vi "Main.vi"(10 "VI":refnum<vi>, 11 "Module Admin":refnum<class "Delacor_lib_QMH_Module Admin.lvclass">) -> ()   [LabVIEW 2019, in "Full User Interface.lvlib"]
doc: "This template is based off of the Queued Message Handler design pattern and the Queued Message Handler project template that ships with LabVIEW.\n\nThe main difference is that the queue is private to this module and communication between modules is performed via Broadcast and Request events.\n\nRequest events are wrapped in public API methods and are handled in the Event Handling Loop (EHL) of this VI. Any module can register for Broadcast events sent by this module. The EHL generates messages based on user interface actions.\n\nThe Message Handling Loop (MHL) processes messages generated by the EHL, or by other messages. The messages are string values, so new messages can be added easily to the Message Cases case structure in the MHL. Each message cluster can also provide an optional value for Message Data, which is a variant that can be converted to whatever message-specific data is required.\n_____\nBased on DQMH Project Template 7.0.1.1316."
uses:
  Full User Interface.lvlib
  <vilib>/Delacor/Delacor QMH/Libraries/Module Admin_class/Delacor_lib_QMH_Module Admin.lvclass
  System.Windows.Forms
  Module Data--cluster.ctl
  Station Config.ctl
  Test Unit/UUT Result.ctl
  <vilib>/Test Bench Framework/Test Executive.lvlibp/TestEngine/TestEngine/TestEngine/Typedefs/Report General.ctl
  <vilib>/Test Bench Framework/Test Executive.lvlibp/TestEngine/TestEngine/TestEngine/Typedefs/TestEngine Cofiguration.ctl
  <vilib>/Test Bench Framework/Test Executive.lvlibp/TestEngine/TestEngine/TestEngine/Typedefs/Local Report Configuration.ctl
  <vilib>/Test Bench Framework/Test Executive.lvlibp/TestEngine/TestEngine/TestEngine/Report Format.ctl
  <vilib>/Test Bench Framework/Test Executive.lvlibp/TestEngine/TestEngine/TestEngine/Typedefs/Database Configuration.ctl
  <vilib>/Delacor/Delacor QMH/Libraries/Message Queue_class/Delacor_lib_QMH_Message Queue.lvclass/Delacor_lib_QMH_Message Queue.ctl
  Change Model Argument--cluster.ctl
  Stop Argument--cluster.ctl
  Launcher Test Unit Argument--cluster.ctl
  Exit Test Unit Argument--cluster.ctl
  Load Seq Argument--cluster.ctl
  Send UUT Result Argument--cluster.ctl
  Send User Message Argument--cluster.ctl
  <vilib>/Delacor/Delacor QMH/Libraries/Module Admin_class/Delacor_lib_QMH_Module Admin.lvclass/Delacor_lib_QMH_Module Admin.ctl
  <vilib>/Delacor/Delacor QMH/Libraries/Message Queue_class/Delacor_lib_QMH_Enqueue Message (Single).vi
  <vilib>/Delacor/Delacor QMH/Libraries/Module Admin_class/Delacor_lib_QMH_Get External Launch.vi
  d3b51c9b-000a-484a-be20-e9c62a2b2a8b.vi
  35dcfc0e-7b8d-49ca-9e41-10d6e4080697.vi
  e5b2156f-1627-4201-8ab9-82cd755b8a05.vi
  8e03fd14-8f50-4f43-832a-65f497bd3936.vi
  2ce45dc2-8b93-4d2c-831c-8eefbe131e90.vi
  7e8d7d5c-7c60-4828-99b6-0f7f76c7f789.vi
  <vilib>/Delacor/Delacor QMH/Libraries/Message Queue_class/Delacor_lib_QMH_Message Queue.lvclass
  Test Unit/Test Unit.lvlib
  <vilib>/Test Bench Framework/Test Executive.lvlibp/TestEngine/TestEngine/TestEngine/Test Engine.lvclass
  <vilib>/Test Bench Framework/Test Executive(API).lvlib
panel:
  in  "Panel":refnum<k24>(container)
  out "error out":errorcluster
  out "Status":string
  in  "Simulate MHL Error":bool
  in  "Simulate EHL Error":bool
types:
  T1 = typedef "Full User Interface.lvlib/Request Events--cluster.ctl" = cluster{"Stop Module":refnum<user-event>, "Show Panel":refnum<user-event>, "Hide Panel":refnum<user-event>, "Get Module Execution Status":refnum<user-event>, "Show Diagram":refnum<user-event>, "Launcher Test Unit":refnum<user-event>, "Exit Test Unit":refnum<user-event>, "Load Seq":refnum<user-event>, "Send UUT Result":refnum<user-event>, "Send User Message":refnum<user-event>, "Change Model":refnum<user-event>}
  T2 = typedef "Full User Interface.lvlib/Module Data--cluster.ctl" = cluster{"Status":string, "menu reference":refnum<k9>, "Key":string, "Config":T3, "UUT Result":refnum<user-event>, "Message":refnum<user-event>, "UserInfo":cluster{"Value":string, "Value":string}, "Configur":T4}
  T3 = typedef "Full User Interface.lvlib/Station Config.ctl" = map{string, map{i32, cluster{"SeqFilename":path, "NumberOfSocket":i32}}}
  T4 = typedef "Test Executive.lvlibp/Test Engine.lvlib/Test Engine.lvclass/TestEngine Cofiguration.ctl" = cluster{"Break on Failure":bool, "Automatically handle TestVI error":cluster{"Enable":bool, "Handle":enum16{"Termination test", "Ignore error"}}, "Local Report Configuration":T5, "Database Configuration":T7, "Ignore breakpoint":bool, "Filter Result":bool}
  T5 = typedef "Test Executive.lvlibp/Test Engine.lvlib/Test Engine.lvclass/Local Report Configuration.ctl" = cluster{"Report Folder Path":path, "Format":T6, "Disable":bool, "Build Date Folder?":bool}
  T6 = typedef "Test Executive.lvlibp/Test Engine.lvlib/Test Engine.lvclass/Report Format.ctl" = enum16{"Excel", "CSV(Tab)", "CSV(,)", "CSV(;)", "TEXT", "HTML"}
  T7 = typedef "Test Executive.lvlibp/Test Engine.lvlib/Test Engine.lvclass/Database Configuration.ctl" = cluster{"Connection String Expression":string, "Microsoft Data Link File":path, "Connection Type":enum16{"Use Connection String Expression", "Use Microsoft Data Link File"}, "Enable":bool}
  T8 = typedef "Full User Interface.lvlib/Change Model Argument--cluster.ctl" = cluster{"Model":string}
  T9 = enum32{"invalid lock state", "Not Locked", "Locked (No Password)", "Password-protected"}
  T10 = typedef "Full User Interface.lvlib/Stop Argument--cluster.ctl" = cluster{"Origin":string, "Exit via Stop Module Req?":bool, "Wait for Module to stop?":bool}
  T11 = typedef "Full User Interface.lvlib/Launcher Test Unit Argument--cluster.ctl" = cluster{"Checkbox":bool}
  T12 = typedef "Full User Interface.lvlib/Exit Test Unit Argument--cluster.ctl" = cluster{"Checkbox":bool}
  T13 = typedef "Full User Interface.lvlib/Load Seq Argument--cluster.ctl" = cluster{"Key":string}
  T14 = typedef "Full User Interface.lvlib/Send UUT Result Argument--cluster.ctl" = cluster{"UUT Result":T15, "Station":i32}
  T15 = typedef "Test Unit.lvlib/UUT Result.ctl" = cluster{"Station":i32, "Socket":i32, "DetailTestResult":string[][], "Report Path":path, "General":T16}
  T16 = typedef "Test Executive.lvlibp/Test Engine.lvlib/Test Engine.lvclass/Report General.ctl" = cluster{"Sequence Path":path, "Serial Number":string, "Test Date Time":timestamp, "UUT Status":string, "Faulty Item":string, "Seconds Executing":dbl}
  T17 = typedef "Full User Interface.lvlib/Send User Message Argument--cluster.ctl" = cluster{"Station ID":i32, "Socket":i32, "UserMessage":string, "MessageData":variant}
  T18 = enum32{"Invalid", "Standard", "Closed", "Hidden", "Minimized", "Maximized"}
  T19 = cluster{"Error":errorcluster, "Additional Information":string, "Module ID":i32, "Module Name":string}
  T20 = cluster{"Module ID":i32, "Origin":string, "Exit via Stop Module Req?":bool, "Wait for Module to stop?":bool}
  T21 = map{i32, cluster{"SeqFilename":path, "NumberOfSocket":i32}}
  T22 = cluster{"SeqFilename":path, "NumberOfSocket":i32}
  T23 = cluster{"Left":i32, "Top":i32, "Right":i32, "Bottom":i32}
  T24 = typedef "LVRectTypeDef.ctl" = cluster{"Left":i16, "Top":i16, "Right":i16, "Bottom":i16}
  T25 = cluster{"Error":errorcluster, "Additional Information":string, "Module Name":string}
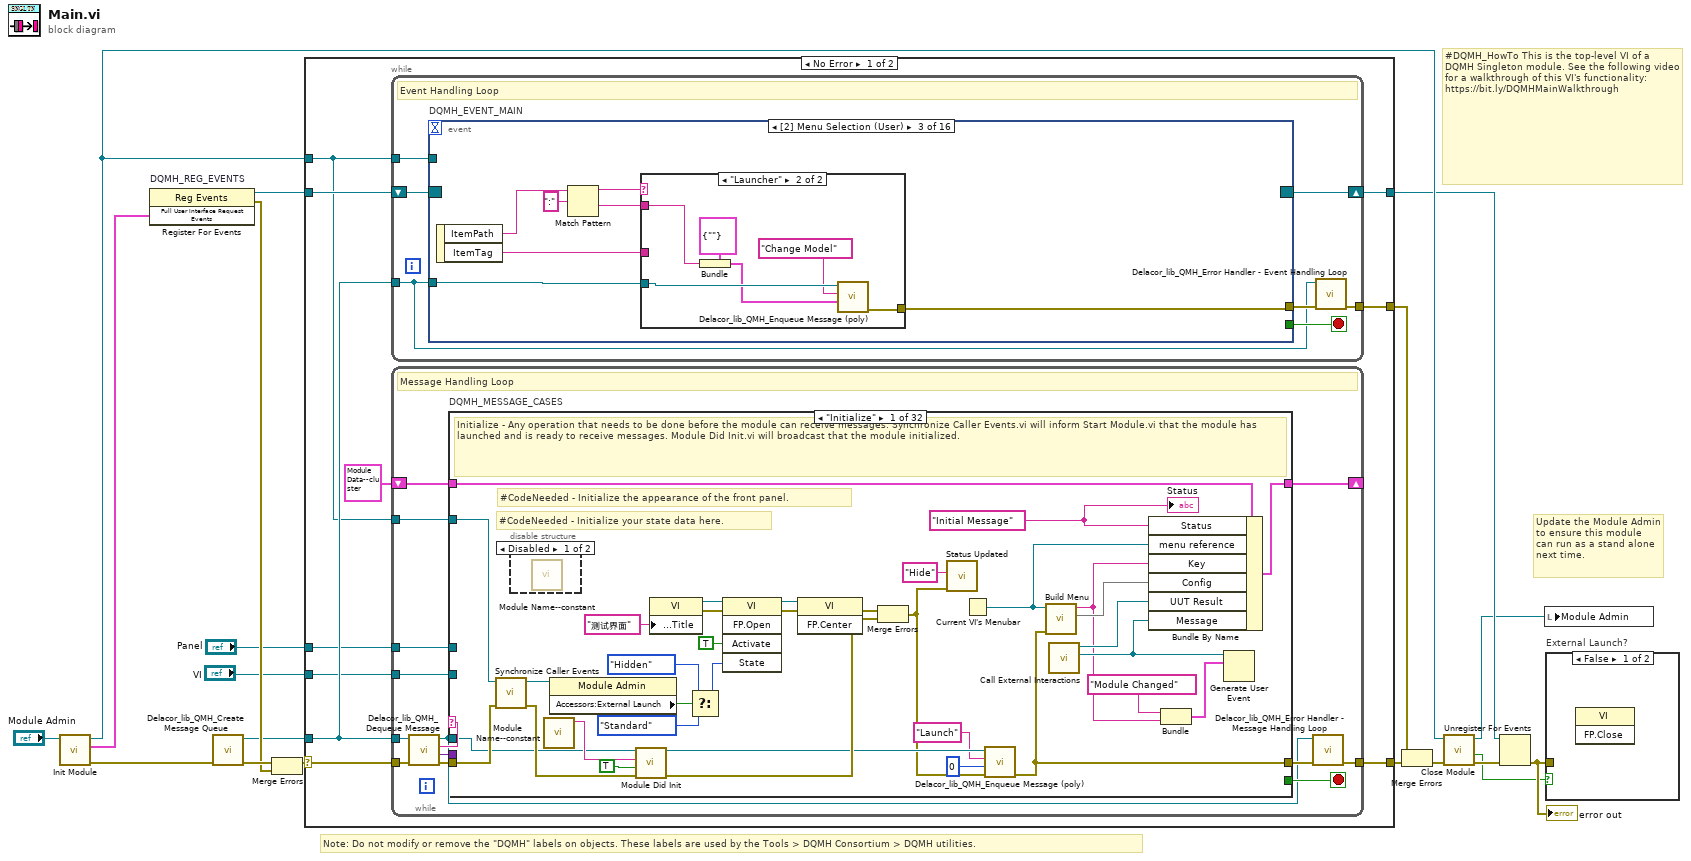
[diagram p0: block diagram]
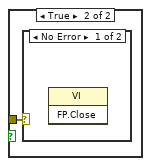
[diagram p2: hidden frame]
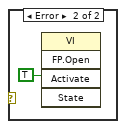
[diagram p3: hidden frame]
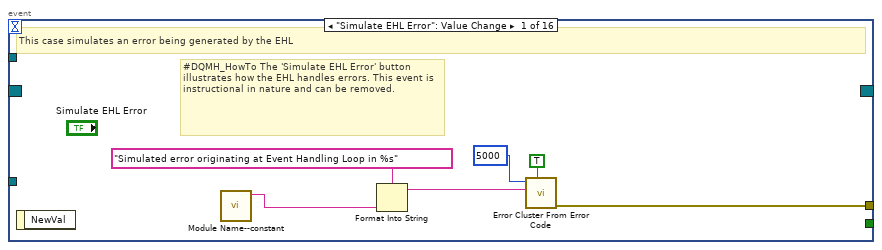
[diagram p4: hidden frame]
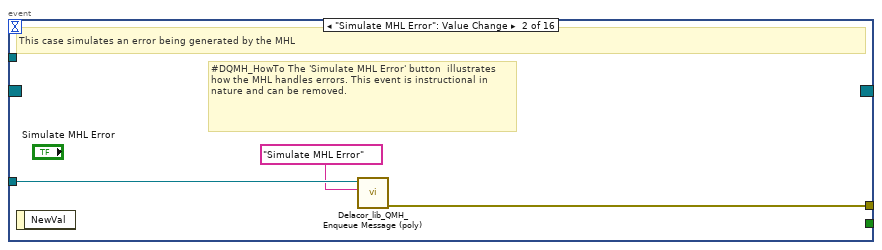
[diagram p5: hidden frame]
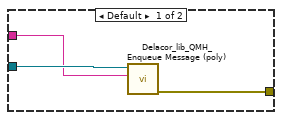
[diagram p6: hidden frame]
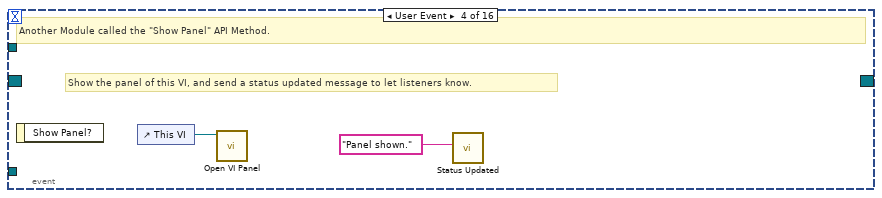
[diagram p7: hidden frame]
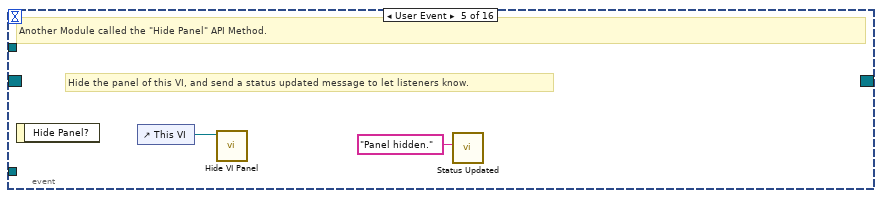
[diagram p8: hidden frame]
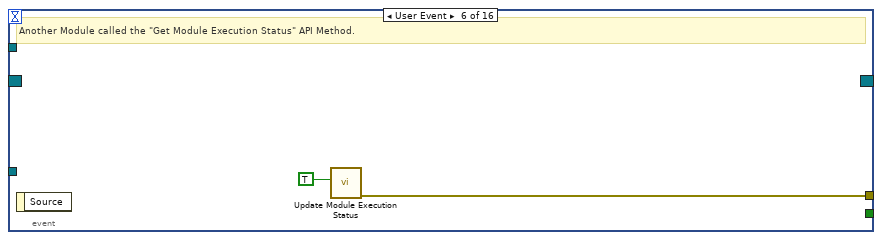
[diagram p9: hidden frame]
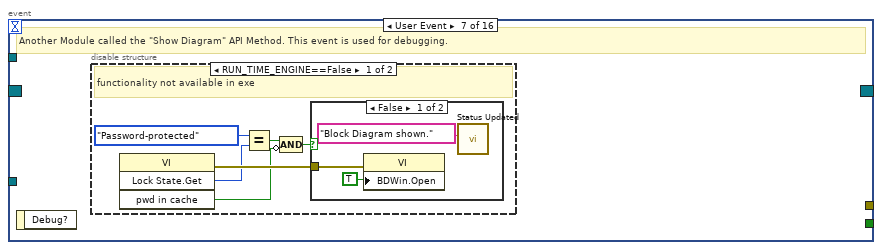
[diagram p10: hidden frame]
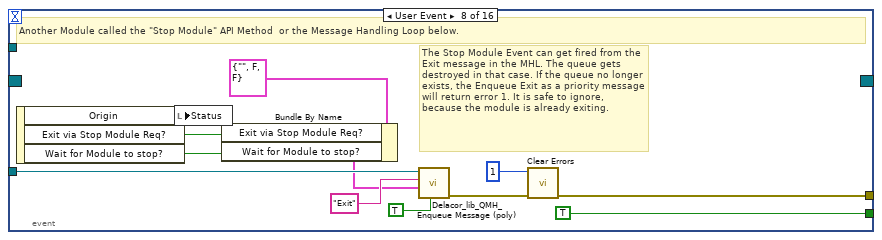
[diagram p13: hidden frame]
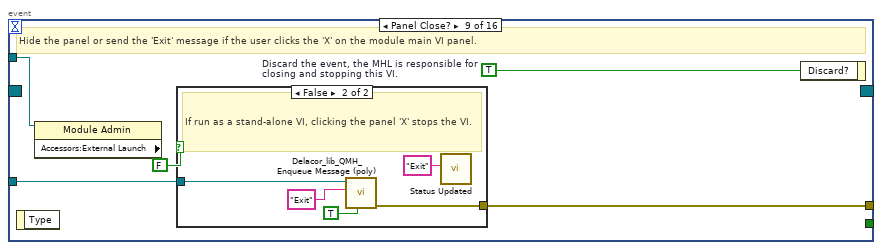
[diagram p14: hidden frame]
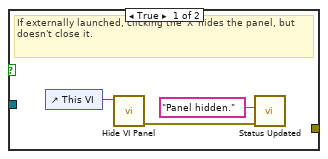
[diagram p15: hidden frame]
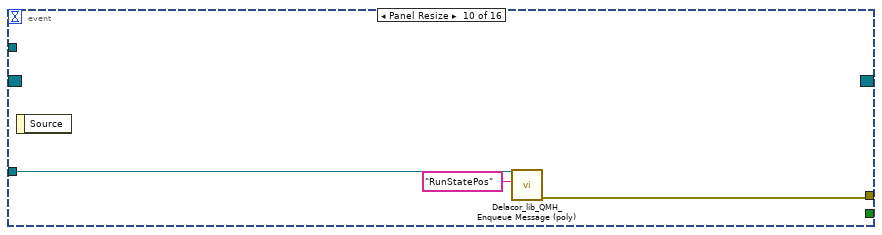
[diagram p16: hidden frame]
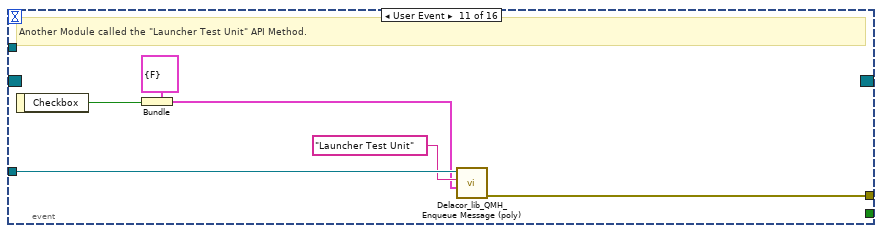
[diagram p17: hidden frame]
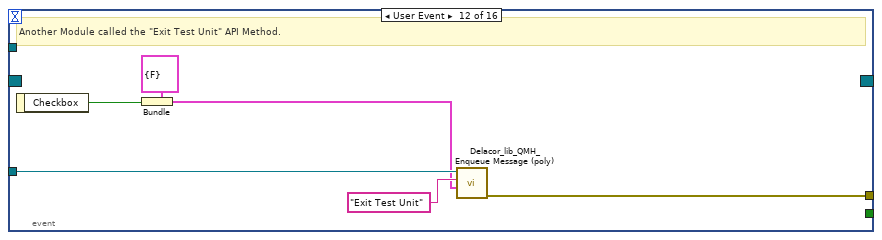
[diagram p18: hidden frame]
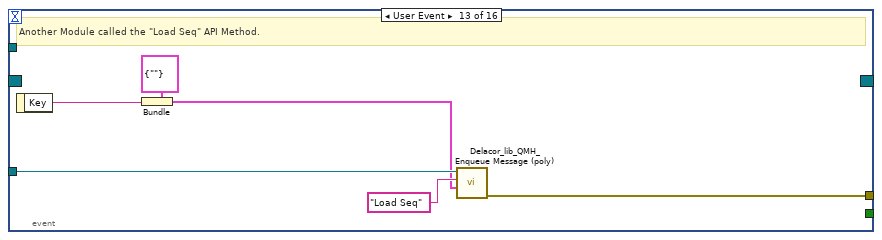
[diagram p19: hidden frame]
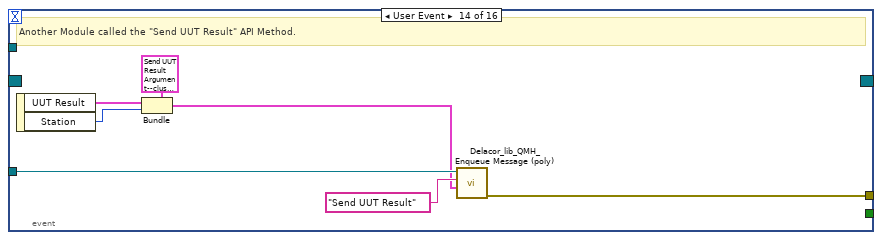
[diagram p20: hidden frame]
diagram:
  # "#DQMH_HowTo This is the top-level VI of a DQMH Singleton module. See the following video for a walkthrough of this VI's functionality: https://bit.ly/DQMHMainWalkthrough"
  # "Note: Do not modify or remove the \"DQMH\" labels on objects. These labels are used by the Tools > DQMH Consortium > DQMH utilities."
  # "Update the Module Admin to ensure this module can run as a stand alone next time."
  n1 = call "Init Module.vi"("Singleton Module Admin in"="Module Admin") -> ("error out"=w18:errorcluster, "Full User Interface Request Events"=w7:T1, "Singleton Module Admin out"=w10:refnum<class "Delacor_lib_QMH_Module Admin.lvclass">)  [unwired: 8 in]
  n2 = register-events "DQMH_REG_EVENTS"(w7) -> (reference out=w8:refnum<event-registration>, error out=w11:errorcluster)  [unwired: 2 in]
  n3 = call <vilib>:"Delacor_lib_QMH_Create Message Queue.vi"("error in"=w18) -> ("error out"=w13:errorcluster, "Message Queue"=w6:refnum<class "Delacor_lib_QMH_Message Queue.lvclass">)  [unwired: 9 in]
  n4 = Merge Errors(w13, w11) -> (w12:errorcluster)
  n5 = case shown="No Error" w12 {
    selector: w12 -> [w27 w536]
    tunnel: [w29 w535] -> w19
    tunnel: [w26 w534] -> w9
    tunnel: w8 -> [w24 w534]
    tunnel: w6 -> [w23 w529]
    tunnel: [w28 _] -> w16
    tunnel: w10 -> [w22 w530]
    tunnel: "Panel" -> [w21 _]
    tunnel: "VI" -> [w20 _]
    frame No Error {
      n6 = while {
        tunnel: w23 -> [w30]
        shift-right: [w33] -> w26
        shift-left: w24 -> [w34]
        tunnel: [w35] -> w28
        tunnel: w22 -> [w31]
        stop <- w32 stop-if-true
        # "Event Handling Loop"
        n7 = event "DQMH_EVENT_MAIN" shown="[2] Menu Selection (User)" {
          selector: w34 -> [_ _ _ _ _ _ _ _ _ _ _ _ _ _ _ _]
          dyn-events: [_ _ _ _ _ _ _ _ _ _ _ _ _ _ _ _] -> w33
          timeout: _ -> [_ _ _ _ _ _ _ _ _ _ _ _ _ _ _ _]
          tunnel: [_ _ _ _ _ _ _ TRUE ("Discard?") _ _ _ _ _ _ _ _] -> w32
          tunnel: w30 -> [_ w44 w52 _ _ _ _ w84 w91 w104 w110 w116 w122 w129 w138 w144]
          tunnel: [w42 w45 w50 _ _ w67 _ w87 w93 w103 w105 w111 w117 w123 w134 w139] -> w36
          tunnel: w31 -> [_ _ _ _ _ _ _ _ w90 _ _ _ _ _ _ _]
          event "Simulate EHL Error": Value Change {
            # "#DQMH_HowTo The 'Simulate EHL Error' button  illustrates how the EHL handles errors. This event is instructional in nature and can be removed."
            # "This case simulates an error being generated by the EHL"
            n8 = event-data() -> ()  [unwired: 1 in, 1 out]
            n9 = call "Module Name--constant.vi"() -> ("Module Name"=w39:string)  [unwired: 11 in]
            n10 = Format Into String(format string="Simulated error originating at Event Handling Loop in %s", w39) -> (resulting string=w40:string)  [unwired: 2 in, 1 out]
            n11 = call <vilib>:"Error Cluster From Error Code.vi"("show call chain? (False)"=TRUE, "error message (\"\")"=w40, "error code (0)"=5000) -> ("error out"=w42:errorcluster)  [unwired: 6 in]
          }
          event "Simulate MHL Error": Value Change {
            # "#DQMH_HowTo The 'Simulate MHL Error' button  illustrates how the MHL handles errors. This event is instructional in nature and can be removed."
            # "This case simulates an error being generated by the MHL"
            n12 = event-data() -> ()  [unwired: 1 in, 1 out]
            n13 = call-poly <vilib>:"Delacor_lib_QMH_Enqueue Message (poly).vi"("Message"="Simulate MHL Error", "Message Queue in"=w44) -> ("error out"=w45:errorcluster)  [unwired: 8 in, 1 out]
          }
          event Menu Selection (User) {
            n14 = event-data() -> ("ItemPath"=w49:string, "ItemTag"=w51:string)  [unwired: 1 in]
            n15 = Match Pattern(string=w49, regular expression=":") -> (before substring=w47:string, after substring=w46:string)  [unwired: 1 in, 2 out]
            n16 = case shown="\"Launcher\"" w47 {
              tunnel: w52 -> [w55 w60]
              tunnel: w51 -> [w54 _]
              tunnel: [w53 w61] -> w50
              tunnel: w46 -> [_ w57]
              frame Default {
                n17 = call-poly <vilib>:"Delacor_lib_QMH_Enqueue Message (poly).vi"("Message"=w54, "Message Queue in"=w55) -> ("error out"=w53:errorcluster)  [unwired: 8 in, 1 out]
              }
              frame "Launcher" {
                n18 = Bundle(cluster=T8 {"Model"=""} ("Change Model Argument"), "Model"=w57) -> (w56:T8)
                n19 = call-poly <vilib>:"Delacor_lib_QMH_Enqueue Message (poly).vi"("Message Data"=w56, "Message"="Change Model", "Message Queue in"=w60) -> ("error out"=w61:errorcluster)  [unwired: 7 in, 1 out]
              }
            }
          }
          event User Event {
            # "Show the panel of this VI, and send a status updated message to let listeners know."
            # "Another Module called the \"Show Panel\" API Method."
            n20 = event-data() -> ()  [unwired: 1 in, 1 out]
            n21 = control-ref of="This VI"() -> (w63:refnum<vi>)
            n22 = call "Open VI Panel.vi"("VI"=w63) -> ()  [unwired: 10 in, 1 out]
            n23 = call "Status Updated.vi"("Status"="Panel shown." ("format string")) -> ()  [unwired: 10 in, 1 out]
          }
          event User Event {
            # "Hide the panel of this VI, and send a status updated message to let listeners know."
            # "Another Module called the \"Hide Panel\" API Method."
            n24 = event-data() -> ()  [unwired: 1 in, 1 out]
            n25 = control-ref of="This VI"() -> (w65:refnum<vi>)
            n26 = call "Hide VI Panel.vi"("VI"=w65) -> ()  [unwired: 10 in, 1 out]
            n27 = call "Status Updated.vi"("Status"="Panel hidden." ("format string")) -> ()  [unwired: 10 in, 1 out]
          }
          event User Event {
            # "Another Module called the \"Get Module Execution Status\" API Method."
            n28 = event-data() -> ()  [unwired: 1 in, 1 out]
            n29 = call "Update Module Execution Status.vi"("Running?"=TRUE) -> ("error out"=w67:errorcluster)  [unwired: 10 in]
          }
          event User Event {
            # "Another Module called the \"Show Diagram\" API Method. This event is used for debugging."
            n30 = event-data() -> ()  [unwired: 1 in, 1 out]
            n31 = disable-structure shown="RUN_TIME_ENGINE==False" {
              frame condition #0 (active) {
                # "functionality not available in exe"
                n32 = invoke on="Invoke Node" class="VI" method="Lock State.Get"() -> (error out=w73:errorcluster, "Get Lock State"=w72:T9, "pwd in cache"=w69:bool)  [unwired: 4 in, 1 out]
                n33 = Equal?(x=T9."Password-protected", y=w72) -> (x = y?=w70:bool)
                n34 = Compound Arithmetic op=AND(w70, invert w69) -> (w68:bool)
                n35 = case shown="False" w68 {
                  tunnel: w73 -> [w76 _]
                  frame False {
                    n36 = property on="Property Node" class="VI"(error in=w76, "BDWin.Open"=TRUE ("Block Diagram Window:Open")) -> ()  [unwired: 1 in, 2 out]
                    n37 = call "Status Updated.vi"("Status"="Block Diagram shown." ("format string")) -> ()  [unwired: 10 in, 1 out]
                  }
                  frame True {
                    # "Password-protected VI, and the password is not in the cache. Do not show the diagram."
                  }
                }
              }
              frame condition #1 {
              }
            }
          }
          event User Event {
            # "The Stop Module Event can get fired from the Exit message in the MHL. The queue gets destroyed in that case. If the queue no longer exists, the Enqueue Exit as a priority message will return error 1. It is safe to ignore, because the module is already exiting."
            # "Another Module called the \"Stop Module\" API Method  or the Message Handling Loop below."
            n38 = event-data() -> ("Origin"=w83:string, "Exit via Stop Module Req?"=w79:bool, "Wait for Module to stop?"=w78:bool)  [unwired: 1 in]
            n39 = local write "Status"(w83) -> ()
            n40 = Bundle By Name(cluster=T10 {"Origin"="", "Exit via Stop Module Req?"=FALSE, "Wait for Module to stop?"=FALSE} ("Stop Argument"), "Exit via Stop Module Req?"=w79, "Wait for Module to stop?"=w78) -> (w77:T10)
            n41 = call-poly <vilib>:"Delacor_lib_QMH_Enqueue Message (poly).vi"("Priority Message? (F)"=TRUE, "Message Data"=w77, "Message"="Exit", "Message Queue in"=w84) -> ("error out"=w88:errorcluster)  [unwired: 6 in, 1 out]
            n42 = call <vilib>:"Clear Errors.vi"("error in (no error)"=w88, "specific error code to clear (0: all)"=1) -> ("error out"=w87:errorcluster)  [unwired: 4 in, 1 out]
          }
          event Panel Close? {
            w92 = TRUE  # Discard the event, the MHL is responsible for closing and stopping this VI.
            # "Hide the panel or send the 'Exit' message if the user clicks the 'X' on the module main VI panel."
            n43 = event-data() -> ()  [unwired: 1 in, 1 out]
            n44 = property on="Property Node" class="Module Admin" props=["Accessors:External Launch"](reference=w90) -> ()  [unwired: 1 in, 3 out]
            n45 = case shown="False" FALSE {
              tunnel: w91 -> [_ w100]
              tunnel: [_ w101] -> w93
              frame True {
                # "If externally launched, clicking the 'X' hides the panel, but doesn't close it."
                n46 = control-ref of="This VI"() -> (w96:refnum<vi>)
                n47 = call "Hide VI Panel.vi"("VI"=w96) -> ("error out"=w94:errorcluster)  [unwired: 10 in]
                n48 = call "Status Updated.vi"("error in"=w94, "Status"="Panel hidden." ("format string")) -> ()  [unwired: 9 in, 1 out]
              }
              frame False {
                # "If run as a stand-alone VI, clicking the panel 'X' stops the VI."
                n49 = call-poly <vilib>:"Delacor_lib_QMH_Enqueue Message (poly).vi"("Priority Message? (F)"=TRUE, "Message"="Exit", "Message Queue in"=w100) -> ("error out"=w101:errorcluster)  [unwired: 7 in, 1 out]
                n50 = call "Status Updated.vi"("Status"="Exit") -> ()  [unwired: 10 in, 1 out]
              }
            }
            n51 = event-data ("Event Filter Node")("Discard?"=w92) -> ()  [unwired: 1 in, 1 out]
          }
          event Panel Resize {
            n52 = event-data() -> ()  [unwired: 1 in, 1 out]
            n53 = call-poly <vilib>:"Delacor_lib_QMH_Enqueue Message (poly).vi"("Message"="RunStatePos", "Message Queue in"=w104) -> ("error out"=w103:errorcluster)  [unwired: 8 in, 1 out]
          }
          event User Event {
            # "Another Module called the \"Launcher Test Unit\" API Method."
            n54 = event-data() -> ("Checkbox"=w106:bool)  [unwired: 1 in]
            n55 = Bundle(cluster=T11 {"Checkbox"=FALSE} ("Launcher Test Unit Argument"), "Checkbox"=w106) -> (w107:T11)
            n56 = call-poly <vilib>:"Delacor_lib_QMH_Enqueue Message (poly).vi"("Message Data"=w107, "Message"="Launcher Test Unit", "Message Queue in"=w110) -> ("error out"=w105:errorcluster)  [unwired: 7 in, 1 out]
          }
          event User Event {
            # "Another Module called the \"Exit Test Unit\" API Method."
            n57 = event-data() -> ("Checkbox"=w112:bool)  [unwired: 1 in]
            n58 = Bundle(cluster=T12 {"Checkbox"=FALSE} ("Exit Test Unit Argument"), "Checkbox"=w112) -> (w113:T12)
            n59 = call-poly <vilib>:"Delacor_lib_QMH_Enqueue Message (poly).vi"("Message Data"=w113, "Message"="Exit Test Unit", "Message Queue in"=w116) -> ("error out"=w111:errorcluster)  [unwired: 7 in, 1 out]
          }
          event User Event {
            # "Another Module called the \"Load Seq\" API Method."
            n60 = event-data() -> ("Key"=w118:string)  [unwired: 1 in]
            n61 = Bundle(cluster=T13 {"Key"=""} ("Load Seq Argument"), "Key"=w118) -> (w119:T13)
            n62 = call-poly <vilib>:"Delacor_lib_QMH_Enqueue Message (poly).vi"("Message Data"=w119, "Message"="Load Seq", "Message Queue in"=w122) -> ("error out"=w117:errorcluster)  [unwired: 7 in, 1 out]
          }
          event User Event {
            # "Another Module called the \"Send UUT Result\" API Method."
            n63 = event-data() -> ("UUT Result"=w125:T15, "Station"=w124:i32)  [unwired: 1 in]
            n64 = Bundle(cluster=T14 {"UUT Result"={"Station"=0, "Socket"=0, "DetailTestResult"=[], "Report Path"=path "", "General"={"Sequence Path"=path "", "Serial Number"="", "Test Date Time"=timestamp(0 s since 1904-01-01), "UUT Status"="", "Faulty Item"="", "Seconds Executing"=0.0}}, "Station"=0} ("Send UUT Result Argument"), "UUT Result"=w125, "Station"=w124) -> (w126:T14)
            n65 = call-poly <vilib>:"Delacor_lib_QMH_Enqueue Message (poly).vi"("Message Data"=w126, "Message"="Send UUT Result", "Message Queue in"=w129) -> ("error out"=w123:errorcluster)  [unwired: 7 in, 1 out]
          }
          event User Event {
            # "Another Module called the \"Send User Message\" API Method."
            n66 = event-data() -> ("Station ID"=w133:i32, "Socket"=w132:i32, "UserMessage"=w131:string, "MessageData"=w130:variant)  [unwired: 1 in]
            n67 = Bundle(cluster=T17 {"Station ID"=0, "Socket"=0, "UserMessage"="", "MessageData"=variant(cluster{"Socket":i32, "UserMessage":string, "MessageData":variant} {"Socket"=0, "UserMessage"="", "MessageData"=variant})} ("Send User Message Argument"), "Station ID"=w133, "Socket"=w132, "UserMessage"=w131, "MessageData"=w130) -> (w135:T17)
            n68 = call-poly <vilib>:"Delacor_lib_QMH_Enqueue Message (poly).vi"("Message Data"=w135, "Message"="Send User Message", "Message Queue in"=w138) -> ("error out"=w134:errorcluster)  [unwired: 7 in, 1 out]
          }
          event User Event {
            # "Another Module called the \"Change Model\" API Method."
            n69 = event-data() -> ("Model"=w140:string)  [unwired: 1 in]
            n70 = Bundle(cluster=T8 {"Model"=""} ("Change Model Argument"), "Model"=w140) -> (w141:T8)
            n71 = call-poly <vilib>:"Delacor_lib_QMH_Enqueue Message (poly).vi"("Message Data"=w141, "Message"="Change Model", "Message Queue in"=w144) -> ("error out"=w139:errorcluster)  [unwired: 7 in, 1 out]
          }
        }
        n72 = call-dynamic "Delacor_lib_QMH_Error Handler - Event Handling Loop.vi"("error in"=w36, "Message Queue in"=w30) -> ("dup error in"=w35:errorcluster)  [unwired: 8 in, 1 out]
      }
      n73 = while {
        tunnel: w23 -> [w147]
        shift-right: [w155] -> _
        shift-left: T2 {"Status"="", "menu reference"=refnum, "Key"="", "Config"={}, "UUT Result"=refnum, "Message"=refnum, "UserInfo"={"Value"="", "Value"=""}, "Configur"={"Break on Failure"=FALSE, "Automatically handle TestVI error"={"Enable"=FALSE, "Handle"=enum."Termination test"}, "Local Report Configuration"={"Report Folder Path"=path "", "Format"=enum."Excel", "Disable"=FALSE, "Build Date Folder?"=FALSE}, "Database Configuration"={"Connection String Expression"="", "Microsoft Data Link File"=path "", "Connection Type"=enum."Use Connection String Expression", "Enable"=FALSE}, "Ignore breakpoint"=FALSE, "Filter Result"=FALSE}} ("Data Cluster") -> [w156]
        tunnel: w27 -> [w158]
        tunnel: [w150] -> w29
        tunnel: w22 -> [w151]
        tunnel: w21 -> [w146]
        tunnel: w20 -> [w145]
        stop <- w154 stop-if-true
        # "Message Handling Loop"
        n74 = call-dynamic "Delacor_lib_QMH_Dequeue Message.vi"("error in"=w158, "Message Queue in"=w147) -> ("error out"=w157:errorcluster, "Message Data"=w152:variant, "Message"=w153:string, "Message Queue out"=w148:refnum<class "Delacor_lib_QMH_Message Queue.lvclass">)  [unwired: 6 in]
        n75 = case "DQMH_MESSAGE_CASES" shown="\"Initialize\"" w153 {
          selector: w153 -> [_ _ _ _ _ _ _ _ _ _ _ _ _ _ _ _ _ _ _ _ _ _ _ _ _ _ _ _ _ _ _ w524]
          tunnel: w148 -> [w173 _ w208 w228 w262 _ _ w289 w304 _ _ _ _ _ _ _ _ _ _ w409 _ _ _ _ _ _ _ _ _ w486 w512 _]
          tunnel: w157 -> [w190 w194 w207 w229 w264 w272 w279 w296 w308 w310 w326 w344 w354 w357 w362 w377 w392 w398 w404 w408 w424 w434 w448 w457 w460 w468 w471 w473 w482 w493 w518 w527]
          tunnel: [w170 w194 w206 w226 w260 w269 w276 w288 w305 w309 w318 w343 w353 w356 w361 w376 w391 w399 w403 w419 w423 w433 w447 w456 w459 w468 w471 w473 w481 w489 w513 w528] -> w149
          tunnel: w156 -> [w181 w193 w202 w222 w265 w268 w275 w292 w307 w313 w325 w339 w350 w355 w360 w375 w390 w396 w402 w418 w422 w432 w446 w455 w458 w467 w470 w472 w479 w488 w500 w525]
          tunnel: [w180 w193 w202 w222 w265 w266 w273 w291 w307 w313 w325 w339 w350 w355 w360 w375 w390 w395 w402 w418 w422 w432 w446 w455 w458 w467 w470 w472 w479 w488 w500 w525] -> w155
          tunnel: [_ _ _ _ _ _ _ _ _ _ _ _ _ _ _ _ _ _ _ _ _ _ _ _ _ _ _ _ _ _ w511 _] -> w154
          tunnel: w152 -> [_ _ w205 w236 _ _ _ w295 _ _ w323 w342 w352 _ _ _ _ _ _ _ _ w431 w445 w454 _ _ _ _ _ w487 w510 _]
          tunnel: w151 -> [w182 _ _ _ _ _ _ _ _ _ _ _ _ _ _ _ _ _ _ _ _ _ _ _ _ _ _ _ _ w485 w505 _]
          tunnel: w146 -> [_ _ _ w232 _ _ _ _ _ _ _ _ _ _ _ w373 w386 _ _ _ _ _ _ _ _ _ _ _ _ _ _ _]
          tunnel: w145 -> [_ _ _ _ _ _ _ _ _ _ _ _ _ _ _ _ _ _ _ _ w421 _ _ _ _ _ _ _ _ _ _ _]
          frame "Initialize" {
            w176 = "Initial Message" ("Initial Message")
            # "#CodeNeeded - Initialize the appearance of the front panel."
            # "#CodeNeeded - Initialize your state data here."
            # "Initialize - Any operation that needs to be done before the module can receive messages. Synchronize Caller Events.vi will inform Start Module.vi that the module has launched and is ready to receive messages. Module Did Init.vi will broadcast that the module initialized."
            n76 = call "Synchronize Caller Events.vi"("error in"=w190, "Singleton Module Admin in"=w182) -> ("error out"=w189:errorcluster, "Singleton Module Admin out"=w177:refnum<class "Delacor_lib_QMH_Module Admin.lvclass">)  [unwired: 8 in]
            n77 = disable-structure shown="Disabled" {
              frame Disabled {
                n78 = call "Module Name--constant.vi"() -> ()  [unwired: 11 in, 1 out]
              }
              frame Enabled {
              }
            }
            n79 = call "Module Name--constant.vi"() -> ("Module Name"=w178:string)  [unwired: 11 in]
            n80 = property on="Property Node" class="Module Admin"(reference=w177) -> ("Accessors:External Launch"=w186:bool)  [unwired: 1 in, 2 out]
            n81 = call "Module Did Init.vi"("error in"=w189, "Initialized?"=TRUE, "Origin"=w178) -> ("error out"=w174:errorcluster)  [unwired: 8 in]
            n82 = property on="Property Node" class="VI"("Front Panel.Title"="测试界面" ("Front Panel Window:Title")) -> (reference out=w188:refnum<vi>, error out=w192:errorcluster)  [unwired: 2 in]
            n83 = Select(t=T18."Hidden" ("State"), s=w186, f=T18."Standard" ("State")) -> (s? t:f=w183:T18)
            n84 = invoke on="Invoke Node" class="VI" method="FP.Open"(reference=w188, error in=w192, "Activate"=TRUE ("Activate?"), "State"=w183) -> (reference out=w187:refnum<vi>, error out=w191:errorcluster)  [unwired: 1 in, 3 out]
            n85 = invoke on="Invoke Node" class="VI" method="FP.Center"(reference=w187, error in=w191) -> (error out=w175:errorcluster)  [unwired: 1 in, 2 out]
            n86 = Merge Errors(w175, w174) -> (w164:errorcluster)
            n87 = call "Status Updated.vi"("error in"=w164, "Status"="Hide") -> ()  [unwired: 9 in, 1 out]
            n88 = Current VI's Menubar() -> (w169:refnum<k9>)
            n89 = call-poly <vilib>:"Delacor_lib_QMH_Enqueue Message (poly).vi"("error in"=w164, "Message Data"=0, "Message"="Launch", "Message Queue in"=w173) -> ("error out"=w170:errorcluster)  [unwired: 6 in, 1 out]
            n90 = call "Build Menu.vi"("error in (no error)"=w170, "menu reference"=w169) -> ("Station Config"=w166:T3, "element"=w160:string)  [unwired: 7 in, 1 out]
            n91 = call "Call External Interactions.vi"() -> ("Message"=w161:refnum<user-event>, "UUT Result"=w165:refnum<user-event>)  [unwired: 9 in, 1 out]
            n92 = Bundle By Name(cluster=w181, "Status"=w176, "menu reference"=w169, "Key"=w160, "Config"=w166, "UUT Result"=w165, "Message"=w161) -> (w180:T2)
            n93 = Bundle("Msg"="Module Changed", "element"=w160) -> (w162:cluster{"Msg":string, "element":string})  [unwired: 1 in]
            n94 = Generate User Event(user event=w161, event data cluster=w162) -> ()  [unwired: 2 in, 2 out]
            "Status" <- w176
          }
          frame "---Module Specific---" {
            # "Separator -- The following cases handle messages specific to this Module."
          }
          frame "Launch" {
            # "Separator -- The following cases handle messages specific to this Module."
            n95 = Variant To Data(type=0, Variant=w205) -> (data=w197:i32)  [unwired: 1 in, 1 out]
            n96 = Unbundle By Name(w202) -> ("Config"=w201:T3, "Key"=w200:string)
            n97 = Look In Map(map=w201, key=w200) -> (key not found?=w199:bool, value=w198:T21)  [unwired: 1 in]
            n98 = Equal To 0?(x=w197) -> (x = 0?=w203:bool)
            n99 = Look In Map(map=w198, key=w197) -> (value=w196:T22)  [unwired: 1 in, 1 out]
            n100 = Unbundle(w196) -> ("NumberOfSocket"=w195:i32)  [unwired: 1 out]
            n101 = case shown="False" w199 {
              tunnel: w208 -> [w213 _]
              tunnel: w207 -> [w212 w214]
              tunnel: [w211 w214] -> w206
              tunnel: w203 -> [w210 _]
              tunnel: w195 -> [w209 _]
              frame False {
                n102 = call "Launch Test Unit.vi"("error in"=w212, "Init Module ID"=w210, "Number of socket"=w209, "Message Queue"=w213) -> ("error out"=w211:errorcluster)  [unwired: 7 in]
              }
              frame True {
              }
            }
          }
          frame "Set Paraent" {
            # "Separator -- The following cases handle messages specific to this Module."
            n103 = Unbundle By Name(w222) -> ("Config"=w223:T3, "Key"=w219:string)
            n104 = Variant To Data(type=cluster{"Module ID":i32, "This VI":refnum<vi>} {"Module ID"=0, "This VI"=refnum} ("output cluster"), Variant=w236) -> (data=w234:cluster{"Module ID":i32, "This VI":refnum<vi>})  [unwired: 1 in, 1 out]
            n105 = Look In Map(map=w223, key=w219) -> (value=w221:T21)  [unwired: 1 in, 1 out]
            n106 = Unbundle(w234) -> ("Module ID"=w217:i32, "This VI"=w233:refnum<vi>)
            n107 = Collection Size(1:w221) -> (0:w220:i32)
            n108 = Equal?(x=w217, y=w220) -> (x = y?=w227:bool)
            n109 = call "Get Win Handle.vi"(".NET Refnum in"=w232) -> ("Bounds"=w224:T23, "ToInt32"=w225:i32)  [unwired: 7 in, 2 out]
            n110 = call "Find Windows.vi"("VI reference"=w233) -> ("hWnd"=w231:u32)  [unwired: 9 in, 1 out]
            n111 = Format Into String(format string="Test Unit %d", w217) -> (resulting string=w216:string)  [unwired: 2 in, 1 out]
            n112 = To Long Integer(number=w231) -> (32bit integer=w230:i32)
            n113 = call "Module Did Init.vi"("Initialized?"=TRUE, "Origin"=w216) -> ()  [unwired: 9 in, 1 out]
            n114 = call "SetParent.vi"("hWndNewParent"=w225, "hWndChild"=w230) -> ()  [unwired: 8 in, 2 out]
            n115 = case shown="True" w227 {
              tunnel: w229 -> [w241 w256]
              tunnel: w228 -> [w240 w245]
              tunnel: [w239 w243] -> w226
              tunnel: w225 -> [_ w259]
              tunnel: w224 -> [_ w258]
              tunnel: w217 -> [w237 _]
              tunnel: w219 -> [_ w250]
              frame False {
                n116 = call-poly <vilib>:"Delacor_lib_QMH_Enqueue Message (poly).vi"("error in"=w241, "Message Data"=w237, "Message"="Launch", "Message Queue in"=w240) -> ("error out"=w239:errorcluster)  [unwired: 6 in, 1 out]
              }
              frame True {
                n117 = call "Stall Data Flow.vim"("value in"=w256, "milliseconds to wait"=u32 100) -> ("value out"=w247:errorcluster)  [unwired: 1 out]
                n118 = call "TileWindows.vi"("Front Panel Window:Panel Bounds"=w258, "error in (no error)"=w247, "hWnd"=w259) -> ("error out"=w257:errorcluster)  [unwired: 8 in]
                n119 = call "Stall Data Flow.vim"("value in"=w257, "milliseconds to wait"=u32 100) -> ("value out"=w252:errorcluster)  [unwired: 1 out]
                n120 = call "TitleWindows.vi"("dont initi"=TRUE, "error in"=w252, "TitleWindows"=TRUE, "Module ID"=-1) -> ("error out"=w244:errorcluster)  [unwired: 7 in]
                n121 = call "Stall Data Flow.vim"("value in"=w244, "milliseconds to wait"=u32 100) -> ("value out"=w249:errorcluster)  [unwired: 1 out]
                n122 = call-poly <vilib>:"Delacor_lib_QMH_Enqueue Message (poly).vi"("error in"=w244, "Message"="SetTestUnitConfig", "Message Queue in"=w245) -> ("error out"=w243:errorcluster)  [unwired: 7 in, 1 out]
                n123 = call "Load Seq.vi"("error in"=w249, "Key"=w250) -> ()  [unwired: 9 in, 1 out]
              }
            }
          }
          frame "TestUnitConfig" {
            n124 = call "Config.vi"("Error In"=w264) -> ("Error Out"=w263:errorcluster)  [unwired: 10 in]
            n125 = call-poly <vilib>:"Delacor_lib_QMH_Enqueue Message (poly).vi"("error in"=w263, "Message"="SetTestUnitConfig", "Message Queue in"=w262) -> ("error out"=w260:errorcluster)  [unwired: 7 in, 1 out]
          }
          frame "SetTestUnitConfig" {
            n126 = call "Get Config.vi"("error in (no error)"=w272) -> ("error out"=w271:errorcluster, "Configur"=w267:T4)  [unwired: 9 in]
            n127 = Bundle By Name(cluster=w268, "Configur"=w267) -> (w266:T2)
            n128 = call "Cofiguration.vi"("error in"=w271, "TestEngine Cofiguration"=w267, "Module ID"=-1) -> ("error out"=w269:errorcluster)  [unwired: 8 in]
          }
          frame "StationConfig" {
            n129 = call "Station Config.vi"("error IO"=w279) -> ("error IO 2"=w277:errorcluster)  [unwired: 10 in]
            n130 = Unbundle By Name(w275) -> ("menu reference"=w278:refnum<k9>)
            n131 = call "ReBuild Menu.vi"("error in (no error)"=w277, "menu reference"=w278) -> ("error out"=w276:errorcluster, "Station Config"=w274:T3)  [unwired: 8 in]
            n132 = Bundle By Name(cluster=w275, "Config"=w274) -> (w273:T2)
          }
          frame "Change Model" {
            n133 = Variant To Data(type=T8 {"Model"=""} ("Change Model Argument"), Variant=w295) -> (data=w284:T8)  [unwired: 1 in, 1 out]
            n134 = Unbundle By Name(w292) -> ("menu reference"=w294:refnum<k9>, "Message"=w283:refnum<user-event>)
            n135 = Unbundle By Name(w284) -> ("Model"=w281:string)
            n136 = call "Select Config.vi"("item tag"=w281, "menu reference"=w294) -> ("error out"=w293:errorcluster)  [unwired: 9 in]
            n137 = Bundle("Msg"="Module Changed", "Model"=w281) -> (w280:cluster{"Msg":string, "Model":string})  [unwired: 1 in]
            n138 = Generate User Event(user event=w283, event data cluster=w280) -> ()  [unwired: 2 in, 2 out]
            n139 = call "Get Station Config.vi"() -> ("Station Config"=w286:T3)  [unwired: 10 in, 1 out]
            n140 = Bundle By Name(cluster=w292, "Key"=w281, "Config"=w286) -> (w291:T2)
            n141 = Merge Errors(w293, w296) -> (w290:errorcluster)
            n142 = for {
              tunnel: w289 -> [w301]
              shift-right: [w298] -> w288
              shift-left: w290 -> [w302]
              tunnel: string[] ["Exit Test Unit", "Launcher Test Unit"] -> [w299] mode=indexing
              n143 = call-poly <vilib>:"Delacor_lib_QMH_Enqueue Message (poly).vi"("error in"=w302, "Message"=w299, "Message Queue in"=w301) -> ("error out"=w300:errorcluster)  [unwired: 7 in, 1 out]
              n144 = call "Stall Data Flow.vim"("value in"=w300, "milliseconds to wait"=u32 100) -> ("value out"=w298:errorcluster)  [unwired: 1 out]
            }
          }
          frame "Launcher Test Unit" {
            n145 = call-poly <vilib>:"Delacor_lib_QMH_Enqueue Message (poly).vi"("error in"=w308, "Message Data"=0, "Message"="Launch", "Message Queue in"=w304) -> ("error out"=w305:errorcluster)  [unwired: 6 in, 1 out]
          }
          frame "Exit Test Unit" {
            # "#CodeNeeded\n1. Configure this Message Case for handling the \"Exit Test Unit\" message.\n2. Delete or edit this label when done."
            n146 = call "Stop Module.vi"("error in"=w310, "Wait for Module to stop? (F)"=TRUE, "Module ID"=-1) -> ("error out"=w309:errorcluster)  [unwired: 8 in]
          }
          frame "Load Seq" {
            n147 = Variant To Data(error in=w326, type=T13 {"Key"=""} ("Load Seq Argument"), Variant=w323) -> (data=w321:T13, error out=w324:errorcluster)
            n148 = Unbundle By Name(w321) -> ("Key"=w316:string)
            n149 = call "Get Station Config.vi"() -> ("Station Config"=w320:T3)  [unwired: 10 in, 1 out]
            n150 = Look In Map(map=w320, key=w316) -> (value=w319:T21)  [unwired: 1 in, 1 out]
            n151 = for {
              tunnel: w319 -> [w334] mode=indexing
              shift-right: [w328] -> w317
              shift-left: _ -> [w327]
              n152 = Unbundle(w334) -> ("Station"=w333:i32, "value"=w332:T22)
              n153 = Unbundle(w332) -> ("SeqFilename"=w330:path)  [unwired: 1 out]
              n154 = Increment(x=w333) -> (x+1=w331:i32)
              n155 = call "Load Sequence.vi"("error in"=w327, "Sequence"="Main_Sequence", "File Pathname"=w330, "Module ID"=w331) -> ("error out"=w328:errorcluster)  [unwired: 7 in]
            }
            n156 = Format Into String(format string="Switch Product %s", w316) -> (resulting string=w314:string)  [unwired: 2 in, 1 out]
            n157 = call "Status Updated.vi"("Status"=w314) -> ()  [unwired: 10 in, 1 out]
            n158 = Merge Errors(w317, w324) -> (w318:errorcluster)
          }
          frame "Send UUT Result" {
            n159 = Variant To Data(error in=w344, type=T14 {"UUT Result"={"Station"=0, "Socket"=0, "DetailTestResult"=[], "Report Path"=path "", "General"={"Sequence Path"=path "", "Serial Number"="", "Test Date Time"=timestamp(0 s since 1904-01-01), "UUT Status"="", "Faulty Item"="", "Seconds Executing"=0.0}}, "Station"=0} ("Send UUT Result Argument"), Variant=w342) -> (data=w340:T14, error out=w343:errorcluster)
            n160 = Unbundle By Name(w340) -> ("UUT Result"=w336:T15, "Station"=w337:i32)
            n161 = Unbundle By Name(w339) -> ("UUT Result"=w338:refnum<user-event>)
            n162 = Bundle("Station"=w337, "UUT Result"=w336) -> (w335:cluster{"Station":i32, "UUT Result":T15})  [unwired: 1 in]
            n163 = Generate User Event(user event=w338, event data cluster=w335) -> ()  [unwired: 2 in, 2 out]
          }
          frame "Send User Message" {
            n164 = Variant To Data(error in=w354, type=T17 {"Station ID"=0, "Socket"=0, "UserMessage"="", "MessageData"=variant(cluster{"Socket":i32, "UserMessage":string, "MessageData":variant} {"Socket"=0, "UserMessage"="", "MessageData"=variant})} ("Send User Message Argument"), Variant=w352) -> (data=w348:T17, error out=w353:errorcluster)
            n165 = Unbundle By Name(w350) -> ("Message"=w349:refnum<user-event>)
            n166 = To Variant(anything=w348) -> (Variant=w347:variant)
            n167 = Bundle("Msg"="Client Message", "Variant"=w347) -> (w345:cluster{"Msg":string, "Variant":variant})  [unwired: 1 in]
            n168 = Generate User Event(user event=w349, event data cluster=w345) -> ()  [unwired: 2 in, 2 out]
          }
          frame "---Copy This Frame---" {
            # "Duplicate this frame when creating new messages.  Change this comment in the duplicated frame to describe this message."
            n169 = Merge Errors(w357) -> (w356:errorcluster)
          }
          frame "OpenExtPanel" {
            # "Duplicate this frame when creating new messages.  Change this comment in the duplicated frame to describe this message."
            n170 = Unbundle By Name(w360) -> ("Message"=w359:refnum<user-event>)
            n171 = Generate User Event(user event=w359, event data cluster=cluster{"Msg":string, "Data":variant} {"Msg"="Open Panel", "Data"=variant} ("event data")) -> ()  [unwired: 2 in, 2 out]
            n172 = Merge Errors(w362) -> (w361:errorcluster)
          }
          frame "Vertical" {
            # "Duplicate this frame when creating new messages.  Change this comment in the duplicated frame to describe this message."
            n173 = call "Get Win Handle.vi"(".NET Refnum in"=w373) -> ("error out"=w366:errorcluster, "Bounds"=w371:T23, "ToInt32"=w374:i32)  [unwired: 7 in, 1 out]
            n174 = call "TileWindows.vi"("Front Panel Window:Panel Bounds"=w371, "error in (no error)"=w366, "Vertical?"=TRUE, "hWnd"=w374) -> ("error out"=w367:errorcluster)  [unwired: 7 in]
            n175 = call "Stall Data Flow.vim"("value in"=w367, "milliseconds to wait"=u32 100) -> ("value out"=w365:errorcluster)  [unwired: 1 out]
            n176 = call "TitleWindows.vi"("dont initi"=TRUE, "error in"=w365, "TitleWindows"=TRUE, "Module ID"=-1) -> ("error out"=w363:errorcluster)  [unwired: 7 in]
            n177 = Merge Errors(w363, w377) -> (w376:errorcluster)
          }
          frame "Horizontal" {
            # "Duplicate this frame when creating new messages.  Change this comment in the duplicated frame to describe this message."
            n178 = call "Get Win Handle.vi"(".NET Refnum in"=w386) -> ("error out"=w381:errorcluster, "Bounds"=w387:T23, "ToInt32"=w389:i32)  [unwired: 7 in, 1 out]
            n179 = call "TileWindows.vi"("Front Panel Window:Panel Bounds"=w387, "error in (no error)"=w381, "Vertical?"=FALSE, "hWnd"=w389) -> ("error out"=w382:errorcluster)  [unwired: 7 in]
            n180 = call "Stall Data Flow.vim"("value in"=w382, "milliseconds to wait"=u32 100) -> ("value out"=w380:errorcluster)  [unwired: 1 out]
            n181 = call "TitleWindows.vi"("dont initi"=TRUE, "error in"=w380, "TitleWindows"=TRUE, "Module ID"=-1) -> ("error out"=w378:errorcluster)  [unwired: 7 in]
            n182 = Merge Errors(w378, w392) -> (w391:errorcluster)
          }
          frame "Login" {
            # "Duplicate this frame when creating new messages.  Change this comment in the duplicated frame to describe this message."
            n183 = Unbundle By Name(w396) -> ("menu reference"=w394:refnum<k9>)
            n184 = call <vilib>:"Get User Information.vi"("error in (no error)"=w398) -> ("error out"=w397:errorcluster, "UserInfo"=w393:cluster{"Value":string, "Value":string})  [unwired: 9 in]
            n185 = Bundle By Name(cluster=w396, "UserInfo"=w393) -> (w395:T2)
            n186 = call "Login.vi"("UserInfo"=w393, "menu reference"=w394) -> ()  [unwired: 9 in, 1 out]
            n187 = Merge Errors(w397) -> (w399:errorcluster)
          }
          frame "Logout" {
            # "Duplicate this frame when creating new messages.  Change this comment in the duplicated frame to describe this message."
            n188 = Unbundle By Name(w402) -> ("menu reference"=w401:refnum<k9>)
            n189 = call "Logout.vi"("menu reference"=w401) -> ("Error Out"=w400:errorcluster)  [unwired: 10 in]
            n190 = Merge Errors(w400, w404) -> (w403:errorcluster)
          }
          frame "RunState" {
            w415 = "RunState" ("item tag")
            # "Duplicate this frame when creating new messages.  Change this comment in the duplicated frame to describe this message."
            n191 = Unbundle By Name(w418) -> ("menu reference"=w417:refnum<k9>)
            n192 = Get Menu Item Info(7:w415, 11:w417) -> (3:w416:refnum<k9>, 4:w414:bool)  [unwired: 1 in, 5 out]
            n193 = Not(x=w414) -> (.not. x?=w413:bool)
            n194 = Set Menu Item Info(6:w413, 7:w415, 11:w416) -> ()  [unwired: 4 in, 2 out]
            n195 = Select(t="Show" ("Status"), s=w413, f="Hide") -> (s? t:f=w411:string)
            n196 = call "Status Updated.vi"("Status"=w411) -> ("error out"=w406:errorcluster)  [unwired: 10 in]
            n197 = call-poly <vilib>:"Delacor_lib_QMH_Enqueue Message (poly).vi"("error in"=w408, "Message"="RunStatePos", "Message Queue in"=w409) -> ("error out"=w407:errorcluster)  [unwired: 7 in, 1 out]
            n198 = Merge Errors(w406, w407) -> (w419:errorcluster)
          }
          frame "RunStatePos" {
            # "Duplicate this frame when creating new messages.  Change this comment in the duplicated frame to describe this message."
            n199 = property class="VI"() -> ("Front Panel.WinBounds"=w420:T24)  [unwired: 2 in, 2 out]
            n200 = call "Set Run State Windows Pos.vi"("Front Panel Window:Window Bounds"=w420, "reference"=w421) -> ()  [unwired: 10 in]
            n201 = Merge Errors(w424) -> (w423:errorcluster)
          }
          frame "Status Updated" {
            # "Duplicate this frame when creating new messages.  Change this comment in the duplicated frame to describe this message."
            n202 = Variant To Data(type=cluster{"Status":string, "Module ID":i32} {"Status"="", "Module ID"=0} ("Event Data"), Variant=w431) -> (data=w428:cluster{"Status":string, "Module ID":i32}, error out=w426:errorcluster)  [unwired: 1 in]
            n203 = Unbundle(w428) -> ("Status"=w427:string)  [unwired: 1 out]
            n204 = call "Status Updated.vi"("s"=TRUE, "Status"=w427) -> ("error out"=w425:errorcluster)  [unwired: 9 in]
            n205 = Merge Errors(w425, w426, w434) -> (w433:errorcluster)
          }
          frame "Error Reported" {
            # "Duplicate this frame when creating new messages.  Change this comment in the duplicated frame to describe this message."
            n206 = Variant To Data(type=T19 {"Error"={"status"=FALSE, "code"=0, "source"=""}, "Additional Information"="", "Module ID"=0, "Module Name"=""} ("Event Data"), Variant=w445) -> (data=w443:T19, error out=w437:errorcluster)  [unwired: 1 in]
            n207 = Unbundle By Name(w443) -> ("Error"=w442:errorcluster, "Additional Information"=w441:string, "Module Name"=w440:string)
            n208 = Bundle("Error"=w442, "Additional Information"=w441, "Module Name"=w440) -> (w439:T25)  [unwired: 1 in]
            n209 = call "Error Reported.vi"("DQMH_ARG"=w439, "Boolean"=TRUE, "Error"=errorcluster {"status"=FALSE, "code"=0, "source"=""}) -> ("error out"=w436:errorcluster)  [unwired: 8 in]
            n210 = Merge Errors(w436, w437, w448) -> (w447:errorcluster)
          }
          frame "Module Did Stop" {
            # "Duplicate this frame when creating new messages.  Change this comment in the duplicated frame to describe this message."
            n211 = Variant To Data(type=T20 {"Module ID"=0, "Origin"="", "Exit via Stop Module Req?"=FALSE, "Wait for Module to stop?"=FALSE} ("Event Data"), Variant=w454) -> (data=w452:T20, error out=w450:errorcluster)  [unwired: 1 in]
            n212 = Unbundle By Name(w452) -> ("Origin"=w451:string)
            n213 = call "Module Did Stop.vi"("Origin"=w451) -> ("error out"=w449:errorcluster)  [unwired: 10 in]
            n214 = Merge Errors(w449, w450, w457) -> (w456:errorcluster)
          }
          frame "Update Module Execution Status" {
            # "Duplicate this frame when creating new messages.  Change this comment in the duplicated frame to describe this message."
            n215 = Merge Errors(w460) -> (w459:errorcluster)
          }
          frame "DataQuery" {
            n216 = Unbundle By Name(w467) -> ("Configur.Database Configuration"=w466:T7, "Configur.Database Configuration.Connection String Expression"=w465:string, "Configur.Database Configuration.Microsoft Data Link File"=w464:path)
            n217 = Empty String/Path?(string/path=w465) -> (empty?=w463:bool)
            n218 = Empty String/Path?(string/path=w464) -> (empty?=w462:bool)
            n219 = And(x=w463, y=w462) -> (x .and. y?=w461:bool)
            n220 = case shown="False" w461 {
              tunnel: w466 -> [w469 _]
              frame False {
                n221 = call "DataQuery.vi"("Configur.Database Configuration"=w469) -> ()  [unwired: 10 in, 1 out]
              }
              frame True {
              }
            }
          }
          frame "StatisticalAnalysis" {
          }
          frame "---Exit and Error Handling---" {
            # "Separator - The following cases handle errors and exit messages."
          }
          frame "Simulate MHL Error" {
            # "#DQMH_HowTo The 'Simulate MHL Error' button  illustrates how the MHL handles errors. This event is instructional in nature and can be removed."
            # "Simulate an error occurring at the MHL"
            n222 = call "Module Name--constant.vi"() -> ("Module Name"=w475:string)  [unwired: 11 in]
            n223 = Format Into String(format string="Simulated error originating at Message Handling Loop in %s", w475) -> (resulting string=w476:string)  [unwired: 2 in, 1 out]
            n224 = call <vilib>:"Error Cluster From Error Code.vi"("show call chain? (False)"=TRUE, "error message (\"\")"=w476, "error code (0)"=5001) -> ("error out"=w480:errorcluster)  [unwired: 6 in]
            n225 = Merge Errors(w482, w480) -> (w481:errorcluster)
          }
          frame "Error" {
            # "#CodeRecommended - If the module is running in standalone mode (External Launch = FALSE), this code will pop up an error dialog and call the 'Exit' message if an error occurs. Add more fine-grained error management here."
            # "Error - Check the error message data and respond accordingly. This message is sent by the \"Error Handler\" VIs at the end of each loop in this application."
            n226 = property on="Property Node" class="Module Admin"(reference=w485) -> ("Accessors:External Launch"=w484:bool)  [unwired: 1 in, 2 out]
            n227 = Variant To Data(error in=w493, type=errorcluster {"status"=FALSE, "code"=0, "source"=""} ("error constant"), Variant=w487) -> (data=w483:errorcluster, error out=w491:errorcluster)
            n228 = local write "error out"(w483) -> ()
            n229 = call "Error Reported.vi"("Error"=w483) -> ()  [unwired: 10 in, 1 out]
            n230 = case shown="False" w484 {
              tunnel: [w498 _] -> w490
              tunnel: w486 -> [w496 _]
              tunnel: w483 -> [w497 _]
              frame False {
                n231 = disable-structure shown="DQMH_Disable_SEH==TRUE" {
                  disable-tunnel: w497 -> [w499 _]
                  frame condition #0 (active) {
                    # "If the module is running standalone, then pop up an error dialog and call the \"Exit\" message."
                    n232 = call <vilib>:"Simple Error Handler.vi"("error in (no error)"=w499) -> ()  [unwired: 4 in, 5 out]
                  }
                  frame condition #1 {
                    # "To prevent the Simple Error Handler VI from being loaded (e.g. when deploying to a Real-Time target), add the Conditional Disable Symbol \"DQMH_Disable_SEH\" to your project and set it to TRUE."
                  }
                }
                n233 = call-poly <vilib>:"Delacor_lib_QMH_Enqueue Message (poly).vi"("Priority Message? (F)"=TRUE, "Message"="Exit", "Message Queue in"=w496) -> ("error out"=w498:errorcluster)  [unwired: 7 in, 1 out]
              }
              frame True {
                # "If the module was launched externally, calling the Error Reported broadcast VI is the only action performed by the \"Error\" message. The module's caller can then process the error appropriately."
              }
            }
            n234 = Merge Errors(w491, w490) -> (w489:errorcluster)
          }
          frame "Exit" {
            w509 = 91  # 91: not all Exit messages will have an argument
            w511 = TRUE  # Stop the VI
            # "Release the message queue reference"
            # "#CodeNeeded - Add any required cleanup code here."
            # "Exit - Exit the application."
            n235 = Variant To Data(error in=w518, type=T10 {"Origin"="", "Exit via Stop Module Req?"=FALSE, "Wait for Module to stop?"=FALSE} ("Stop Argument"), Variant=w510) -> (data=w507:T10, error out=w515:errorcluster)
            n236 = call <vilib>:"Clear Errors.vi"("error in (no error)"=w515, "specific error code to clear (0: all)"=w509) -> ("error out"=w517:errorcluster)  [unwired: 4 in, 1 out]
            n237 = control-ref of="This VI"() -> (w506:refnum<vi>)
            n238 = call-dynamic "Delacor_lib_QMH_Release Message Queue.vi"("error in"=w517, "Message Queue"=w512) -> ("error out"=w516:errorcluster)  [unwired: 9 in]
            n239 = call "Handle Exit.vi"("Stop Argument"=w507, "Admin in"=w505, "VI reference"=w506) -> ("error out"=w514:errorcluster)  [unwired: 7 in, 1 out]
            n240 = Merge Errors(w516, w514) -> (w513:errorcluster)
            n241 = Unbundle By Name(w500) -> ("Message"=w502:refnum<user-event>)
            n242 = call "Error Reported.vi"("Error"=w513) -> ()  [unwired: 10 in, 1 out]
            n243 = call "Stop Module.vi"("Wait for Module to stop? (F)"=TRUE, "Module ID"=-1) -> ()  [unwired: 9 in, 1 out]
            n244 = Generate User Event(user event=w502, event data cluster=cluster{"Msg":string, "Data":variant} {"Msg"="Exit", "Data"=variant} ("event data")) -> ()  [unwired: 2 in, 2 out]
          }
          frame Default {
            # "'Default' case only runs if there is a message that isn't defined in any of the other cases.  Output a programming error."
            n245 = call "Module Name--constant.vi"() -> ("Module Name"=w523:string)  [unwired: 11 in]
            n246 = Format Into String(format string="The invalid message string \"%s\" was received in the Message Handling Loop for module \"%s\".", w524, w523) -> (resulting string=w519:string)  [unwired: 2 in, 1 out]
            n247 = call <vilib>:"Error Cluster From Error Code.vi"("show call chain? (False)"=TRUE, "error message (\"\")"=w519, "error code (0)"=1) -> ("error out"=w526:errorcluster)  [unwired: 6 in]
            n248 = Merge Errors(w527, w526) -> (w528:errorcluster)
          }
        }
        n249 = call-dynamic "Delacor_lib_QMH_Error Handler - Message Handling Loop.vi"("error in"=w149, "Message Queue in"=w148) -> ("dup error in"=w150:errorcluster)  [unwired: 8 in, 1 out]
      }
    }
    frame Error {
      # "Synchronize Caller Events.vi will inform Start Module.vi that the module has launched and will let the code calling Start Module.vi register for broadcasts and would permit the caller receive the broadcast that an error occurred at launch time."
      n250 = call-dynamic "Delacor_lib_QMH_Release Message Queue.vi"("error in"=w536, "Message Queue"=w529) -> ("error out"=w535:errorcluster)  [unwired: 9 in]
      n251 = call "Synchronize Caller Events.vi"("Singleton Module Admin in"=w530) -> ("error out"=w537:errorcluster)  [unwired: 9 in, 1 out]
      n252 = call "Module Name--constant.vi"() -> ("Module Name"=w533:string)  [unwired: 11 in]
      n253 = Format Into String(format string="An error occurred during initialization. %s is no longer running.", w533) -> (resulting string=w531:string)  [unwired: 2 in, 1 out]
      n254 = Merge Errors(w535, w537) -> (w538:errorcluster)
      n255 = call "Error Reported.vi"("Additional Information"=w531, "Error"=w538) -> ()  [unwired: 9 in, 1 out]
    }
  }
  n256 = Merge Errors(w16, w19) -> (w15:errorcluster)
  n257 = call "Close Module.vi"("error in"=w15, "Module Admin in"=w10) -> ("error out"=w17:errorcluster, "External Launch"=w3:bool, "Module Admin out"=w4:refnum<class "Delacor_lib_QMH_Module Admin.lvclass">)  [unwired: 7 in]
  n258 = Unregister For Events(event registration refnum=w9, error in=w17) -> (error out=w14:errorcluster)
  "error out" <- w14
  n259 = local write "Module Admin"(w4) -> ()
  n260 = case "External Launch?" shown="False" w3 {
    tunnel: w14 -> [_ w539]
    frame False {
      n261 = invoke on="Invoke Node" class="VI" method="FP.Close"() -> ()  [unwired: 3 in, 3 out]
    }
    frame True {
      n262 = case shown="No Error" w539 {
        frame No Error {
          n263 = invoke on="Invoke Node" class="VI" method="FP.Close"() -> ()  [unwired: 3 in, 3 out]
        }
        frame Error {
          n264 = invoke on="Invoke Node" class="VI" method="FP.Open"("Activate"=TRUE ("Activate?")) -> ()  [unwired: 4 in, 5 out]
        }
      }
    }
  }
